vi "CAENHV Get Sys Prop Info.vi"(8 "error in (no error)":errorcluster, 10 "PropName":string, 11 "handle":i32) -> (0 "error out":errorcluster, 2 "PropType":T1, 3 "PropMode":T2)   [LabVIEW 2018, in "CAENHVWrapper.lvlib"]
doc: "CAENHVLIB_API CAENHVRESULT CAENHV_GetSysPropInfo(int handle, \n const char *PropName, unsigned *PropMode, unsigned *PropType);"
uses:
  <instrlib>/CAENHVWrapper/CAENHVWrapper.lvlib
  <instrlib>/CAENHVWrapper/Types/SYSPROP_MODE.ctl
  <instrlib>/CAENHVWrapper/Types/SYSPROP_TYPE.ctl
  <instrlib>/CAENHVWrapper/VIs/CAENHVWrapper.dll
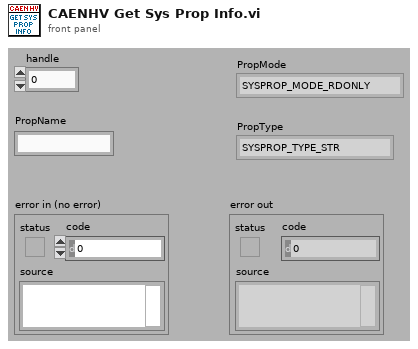
[diagram p1: front panel]
types:
  T1 = typedef "CAENHVWrapper.lvlib/SYSPROP_TYPE.ctl" = enum32{"SYSPROP_TYPE_STR", "SYSPROP_TYPE_REAL", "SYSPROP_TYPE_UINT2", "SYSPROP_TYPE_UINT4", "SYSPROP_TYPE_INT2", "SYSPROP_TYPE_INT4", "SYSPROP_TYPE_BOOLEAN"}
  T2 = typedef "CAENHVWrapper.lvlib/SYSPROP_MODE.ctl" = enum32{"SYSPROP_MODE_RDONLY", "SYSPROP_MODE_WRONLY", "SYSPROP_MODE_RDWR"}
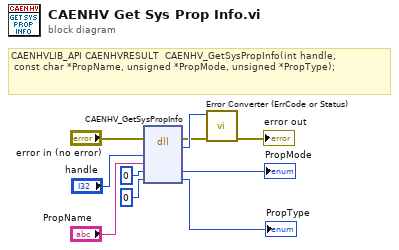
[diagram p0: block diagram]
diagram:
  # "CAENHVLIB_API CAENHVRESULT  CAENHV_GetSysPropInfo(int handle, \n const char *PropName, unsigned *PropMode, unsigned *PropType);"
  n1 = dll-call lib="C:/Program Files (x86)/National Instruments/LabVIEW 2018/instr.lib/CAENHVWrapper/VIs/CAENHVWrapper.*" fn="CAENHV_GetSysPropInfo"(error in="error in (no error)", "handle"="handle", "PropName"="PropName", "PropMode"=u32 0, "PropType"=u32 0) -> (error out=w2:errorcluster, w3:i32, "PropMode"=→"PropMode":u32, "PropType"=→"PropType":u32)  [unwired: 4 in, 1 out]
  n2 = call <instrlib>:"Error Converter (ErrCode or Status).vi"("error in (no error)"=w2, "error code"=w3) -> ("error out"=→"error out":errorcluster)  [unwired: 9 in]
